vi "Get DIO Channel Name.vi"(8 "Error In":errorcluster, 10 "DIO Pins":u8[](array[numeric])) -> (0 "Error Out":errorcluster, 2 "DIO Channels":string[](array[string]))   [LabVIEW 2011, in "LVH-LINX.lvlib" / "myRIO.lvlib"]
uses:
  myRIO.lvlib
  Type Defs/DIO Channel.ctl
panel:
  in  "DIO Channel Enum":T1
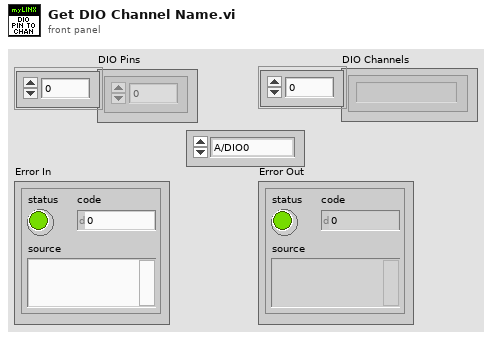
[diagram p1: front panel]
types:
  T1 = typedef "LVH-LINX.lvlib/myRIO.lvlib/DIO Channel.ctl" = enum8{"A/DIO0", "A/DIO1", "A/DIO2", "A/DIO3", "A/DIO4", "A/DIO5", "A/DIO6", "A/DIO7", "A/DIO8", "A/DIO9", "A/DIO10", "A/DIO11", "A/DIO12", "A/DIO13", "A/DIO14", "A/DIO15", "B/DIO0", "B/DIO1", "B/DIO2", "B/DIO3", "B/DIO4", "B/DIO5", "B/DIO6", "B/DIO7", "B/DIO8", "B/DIO9", "B/DIO10", "B/DIO11", "B/DIO12", "B/DIO13", "B/DIO14", "B/DIO15", "C/DIO0", "C/DIO1", "C/DIO2", "C/DIO3", "C/DIO4", "C/DIO5", "C/DIO6", "C/DIO7"}
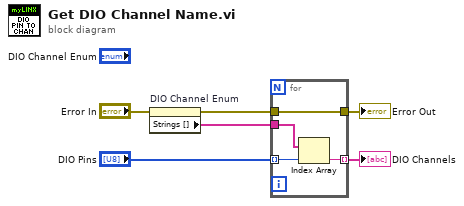
[diagram p0: block diagram]
diagram:
  n1 = property on="DIO Channel Enum" class="Enum (strict)"(error in="Error In") -> (error out=w4:errorcluster, "Strings []"=w3:string[])  [unwired: 1 in, 1 out]
  n2 = for {
    tunnel: [w10] -> w5
    tunnel: w4 -> [w10]
    tunnel: w3 -> [w9]
    tunnel: "DIO Pins" -> [w8] mode=indexing
    tunnel: [w7] -> w1 mode=indexing
    n3 = Index Array(array=w9, index=w8) -> (element=w7:string)
  }
  "Error Out" <- w5
  "DIO Channels" <- w1
